vi "CreateFolder.vi"(11 "path (use dialog)":path=path "C:/Users/Public/Documents/Data") -> (3 "created path":path)   [LabVIEW 2026]
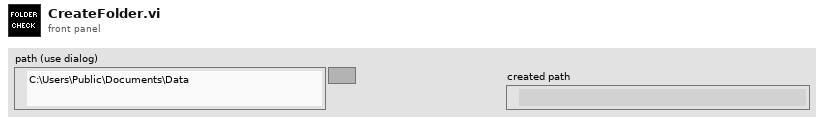
[diagram p1: front panel]
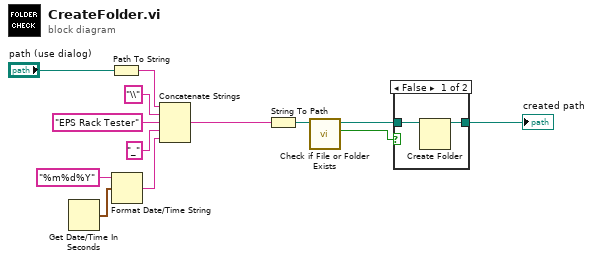
[diagram p0: block diagram]
diagram:
  n1 = Get Date/Time In Seconds() -> (seconds since 1Jan1904=w12:timestamp)
  n2 = Path To String(path="path (use dialog)") -> (string=w9:string)
  n3 = Format Date/Time String(time format string (%c)="%m%d%Y", seconds (now)=w12) -> (date/time string=w8:string)  [unwired: 1 in]
  n4 = Concatenate Strings(w9, "\\" ("string"), "EPS Rack Tester" ("string"), "_" ("string"), w8) -> (w5:string)
  n5 = String To Path(string=w5) -> (path=w3:path)
  n6 = call <vilib>:"Check if File or Folder Exists.vi"("path"=w3) -> ("file or folder exists?"=w1:bool, "dup path"=w2:path)  [unwired: 8 in, 1 out]
  n7 = case shown="False" w1 {
    tunnel: w2 -> [w15 w16]
    tunnel: [w14 w16] -> w4
    frame False {
      n8 = Create Folder(path (use dialog)=w15) -> (created path=w14:path)  [unwired: 2 in, 2 out]
    }
    frame True {
    }
  }
  "created path" <- w4
